vi "To bytes.vi"(3 "MsgPackExt in":refnum<class "MsgPackExt.lvclass">) -> (1 "Array":u8[](array[numeric]))   [LabVIEW 2020, in "MessagePack.lvlib" / "MsgPackExt.lvclass"]
uses:
  MsgPackExt.lvclass
  MsgPackExt.lvclass/MsgPackExt.ctl
  MessagePack.lvlib
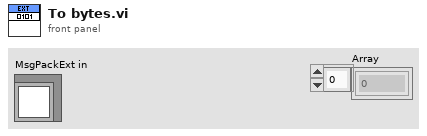
[diagram p1: front panel]
types:
  T1 = typedef "MessagePack.lvlib/MsgPack Object Types.ctl" = enum16{"UNSUPPORTED", "POSINT", "NEGINT", "FIXMAP", "FIXARRAY", "FIXSTR", "NIL", "FALSE", "TRUE", "BIN8", "BIN16", "BIN32", "EXT8", "EXT16", "EXT32", "FLOAT32", "FLOAT64", "UINT8", "UINT16", "UINT32", "UINT64", "INT8", "INT16", "INT32", "INT64", "FIXEXT1", "FIXEXT2", "FIXEXT4", "FIXEXT8", "FIXEXT16", "STR8", "STR16", "STR32", "ARRAY16", "ARRAY32", "MAP16", "MAP32"}
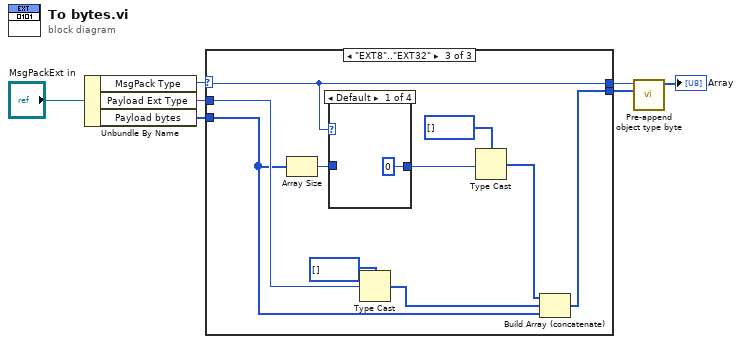
[diagram p0: block diagram]
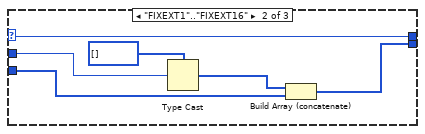
[diagram p3: hidden frame]
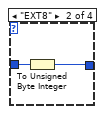
[diagram p4: hidden frame]
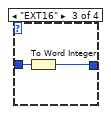
[diagram p5: hidden frame]
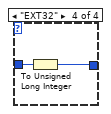
[diagram p6: hidden frame]
diagram:
  n1 = Unbundle By Name("MsgPackExt in") -> ("MsgPack Type"=w6:T1, "Payload Ext Type"=w5:i8, "Payload bytes"=w4:u8[])
  n2 = case shown="\"EXT8\"..\"EXT32\"" w6 {
    selector: w6 -> [_ w8 w19]
    tunnel: w5 -> [_ w12 w22]
    tunnel: w4 -> [_ w11 w20]
    tunnel: [_ w9 w21] -> w3
    tunnel: [_ w8 w19] -> w2
    frame Default {
    }
    frame "FIXEXT1".."FIXEXT16" {
      n3 = Type Cast(type=u8[] [] ("encoded bytes"), x=w12) -> (*(type *) &x=w10:u8[])
      n4 = Build Array (concatenate)(w10, w11) -> (w9:u8[])
    }
    frame "EXT8".."EXT32" {
      n5 = Array Size(array=w20) -> (size(s)=w17:i32)
      n6 = case shown="Default" w19 {
        tunnel: w17 -> [_ w26 w28 w30]
        tunnel: [u32 0 w25 w27 w29] -> w16
        frame Default {
        }
        frame "EXT8" {
          n7 = To Unsigned Byte Integer(number=w26) -> (unsigned 8bit integer=w25:u8)
        }
        frame "EXT16" {
          n8 = To Word Integer(number=w28) -> (16bit integer=w27:i16)
        }
        frame "EXT32" {
          n9 = To Unsigned Long Integer(number=w30) -> (unsigned 32bit integer=w29:u32)
        }
      }
      n10 = Type Cast(type=u8[] [] ("encoded bytes"), x=w22) -> (*(type *) &x=w14:u8[])
      n11 = Type Cast(type=u8[] [] ("encoded bytes"), x=w16) -> (*(type *) &x=w15:u8[])
      n12 = Build Array (concatenate)(w15, w14, w20) -> (w21:u8[])
    }
  }
  n13 = call "Pre-append object type byte.vi"("bytes in"=w3, "Object type"=w2) -> ("encoded bytes"=→"Array":u8[])  [unwired: 8 in, 1 out]
